vi "IntakeGetHaveNote.vi"() -> (3 "IntakeHaveNote":bool)   [LabVIEW 2023]
uses:
  IntakeGlobal.vi
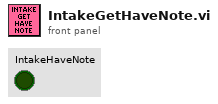
[diagram p1: front panel]
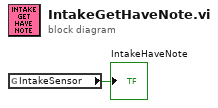
[diagram p0: block diagram]
diagram:
  n1 = global read "IntakeGlobal.vi" "IntakeSensor"() -> (→"IntakeHaveNote":bool)
